vi "DataProcessorRAW.vi"(5 "FPGA in":refnum<queue>, 8 "Queue in":refnum<queue>) -> ()   [LabVIEW 2019, in "FPGA.lvlib"]
uses:
  FPGA.lvlib
  FPGA.ctl
  <vilib>/Analysis/baseanly.llb/Mean (DBL).vi
  <vilib>/Analysis/1siggen.llb/Ramp Pattern by Samples.vi
  ResultSweep.vi
  <vilib>/Analysis/NI_AALBase.lvlib
panel:
  in  "Save raw data":bool
  in  "Output from ADC (SW[9])":bool=TRUE
  in  "autoscale output signal":bool=TRUE
  out "Raw Data":ext[][](graph)
  in  "n. of steps":u32
  in  "Freq. slice start":dbl=10000.0
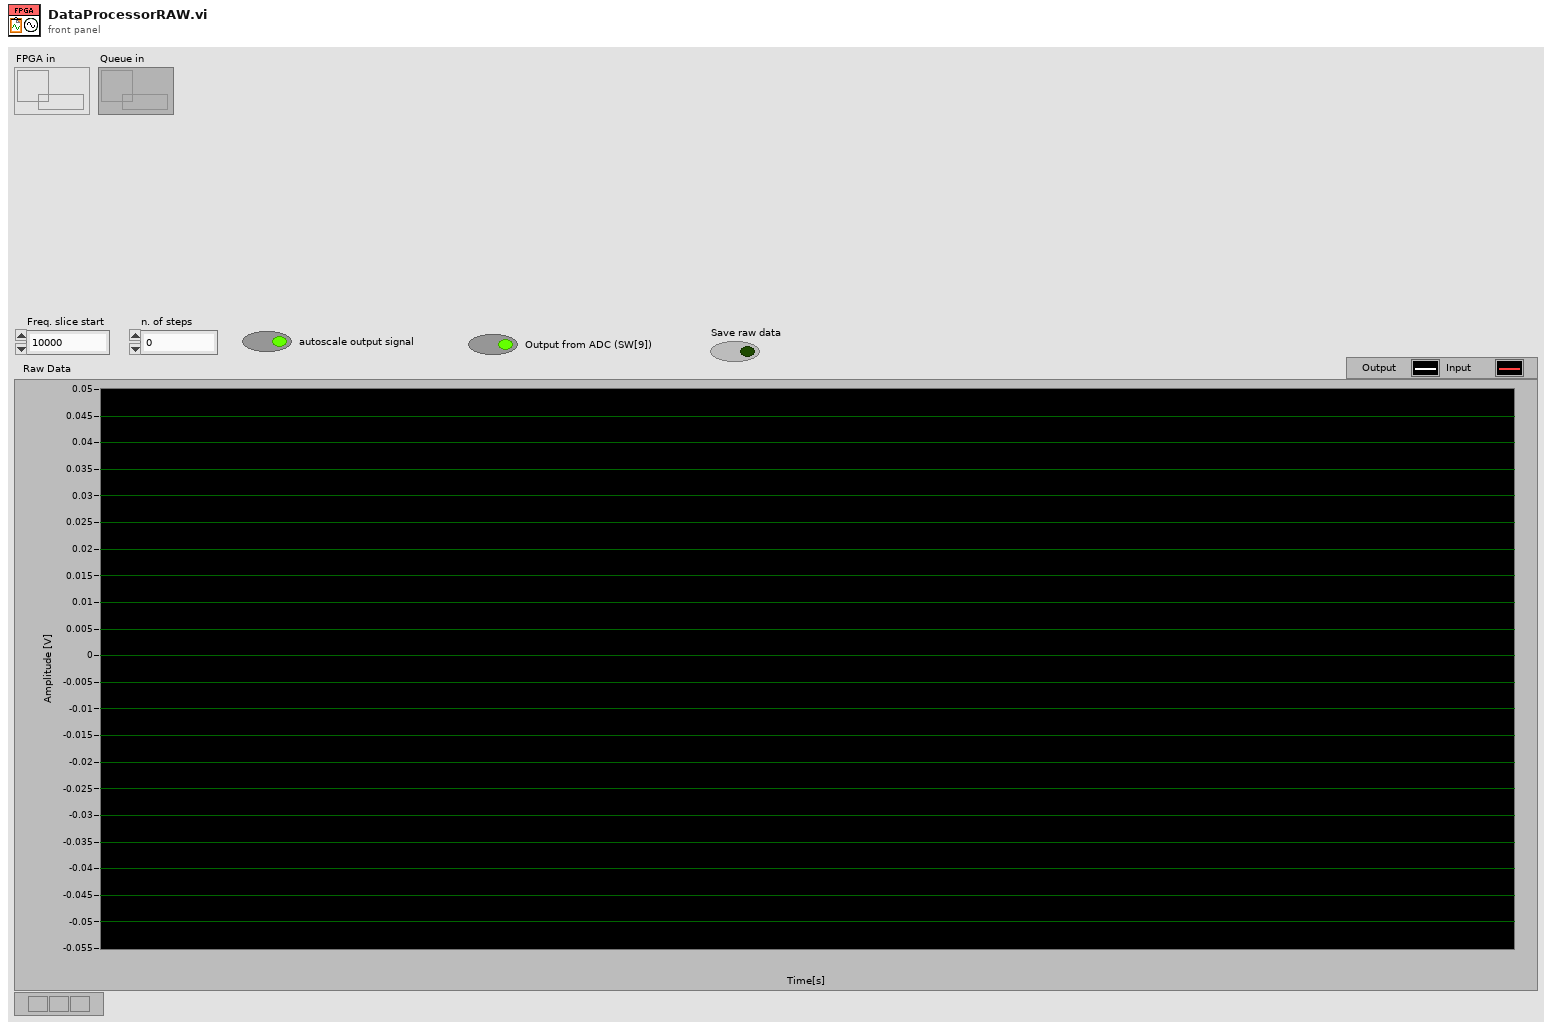
[diagram p1: front panel]
types:
  T1 = typedef "FPGA.lvlib/FPGA.ctl" = cluster{"Start freq. [Hz]":dbl, "Sweep duration [s]":dbl, "Freq. step [Hz]":dbl, "DAC Sample Rate":dbl, "ADC Sample Rate":dbl, "CMD port":u16, "DFAST port":u16, "CMD ID":refnum<k16>, "DFAST ID":refnum<k16>, "CMD error out":errorcluster, "FPGA IP":string, "DFAST error out ":errorcluster, "Stop freq. [Hz]":dbl, "Discrete sweep":bool, "Initial NCO":u32, "Difference NCO":i32, "step NCO":i64, "Final NCO":u32, "clocks for step":u32, "demodulation":bool, "NCO Phase Precision":u32, "NCO Sample Rate":dbl, "Time for step [s]":dbl, "NCO freq. resolution":dbl, "Sweep speed [Hz/s]":dbl, "Connected":bool, "Slew Rate [V/us]":dbl, "Parameters_ok":bool, "Amplitude [mVpp]":dbl, "Scale Factor":fxp<+,16,0>, "Acquiring":bool, "DAC-ADC Latency":u16, "Digital Gain":i32, "Number of steps":i32, "Averaging preferred":bool, "Filter Order":u32, "Settling":enum16{"99%", "99,9%"}}
  T2 = cluster{"Name":string, "Color":u32, "Style":u8, "Point Style":u8, "Name Visible":bool, "Allow Drag":bool, "Cursor Mode":u32, "Plot":i32, "Index":i32, "Position":cluster{"X":dbl, "Y":dbl}, "X Scale":u32, "Y Scale":u32, "Watch Plots":i32[], "Watch All Plots":bool, "Plot Area":i32, "Label Offset":cluster{"X":dbl, "Y":dbl}}
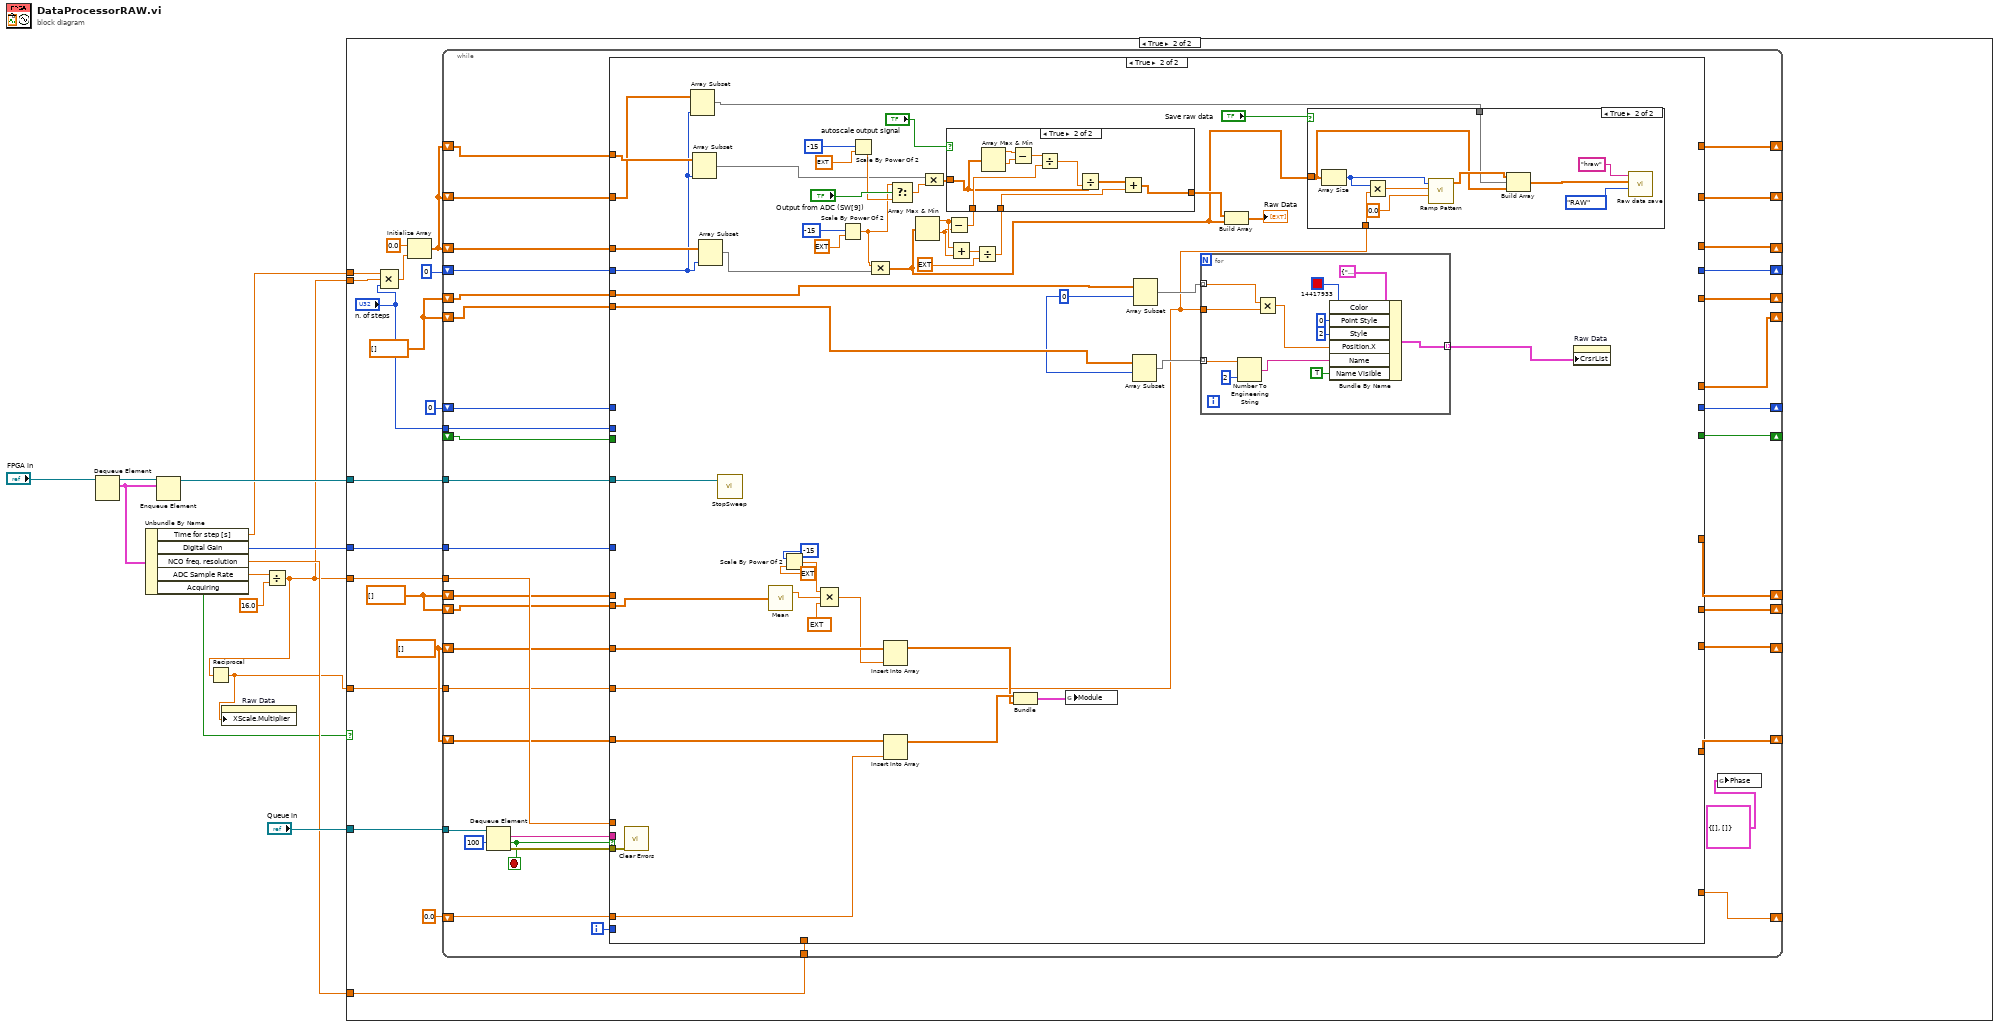
[diagram p0: block diagram]
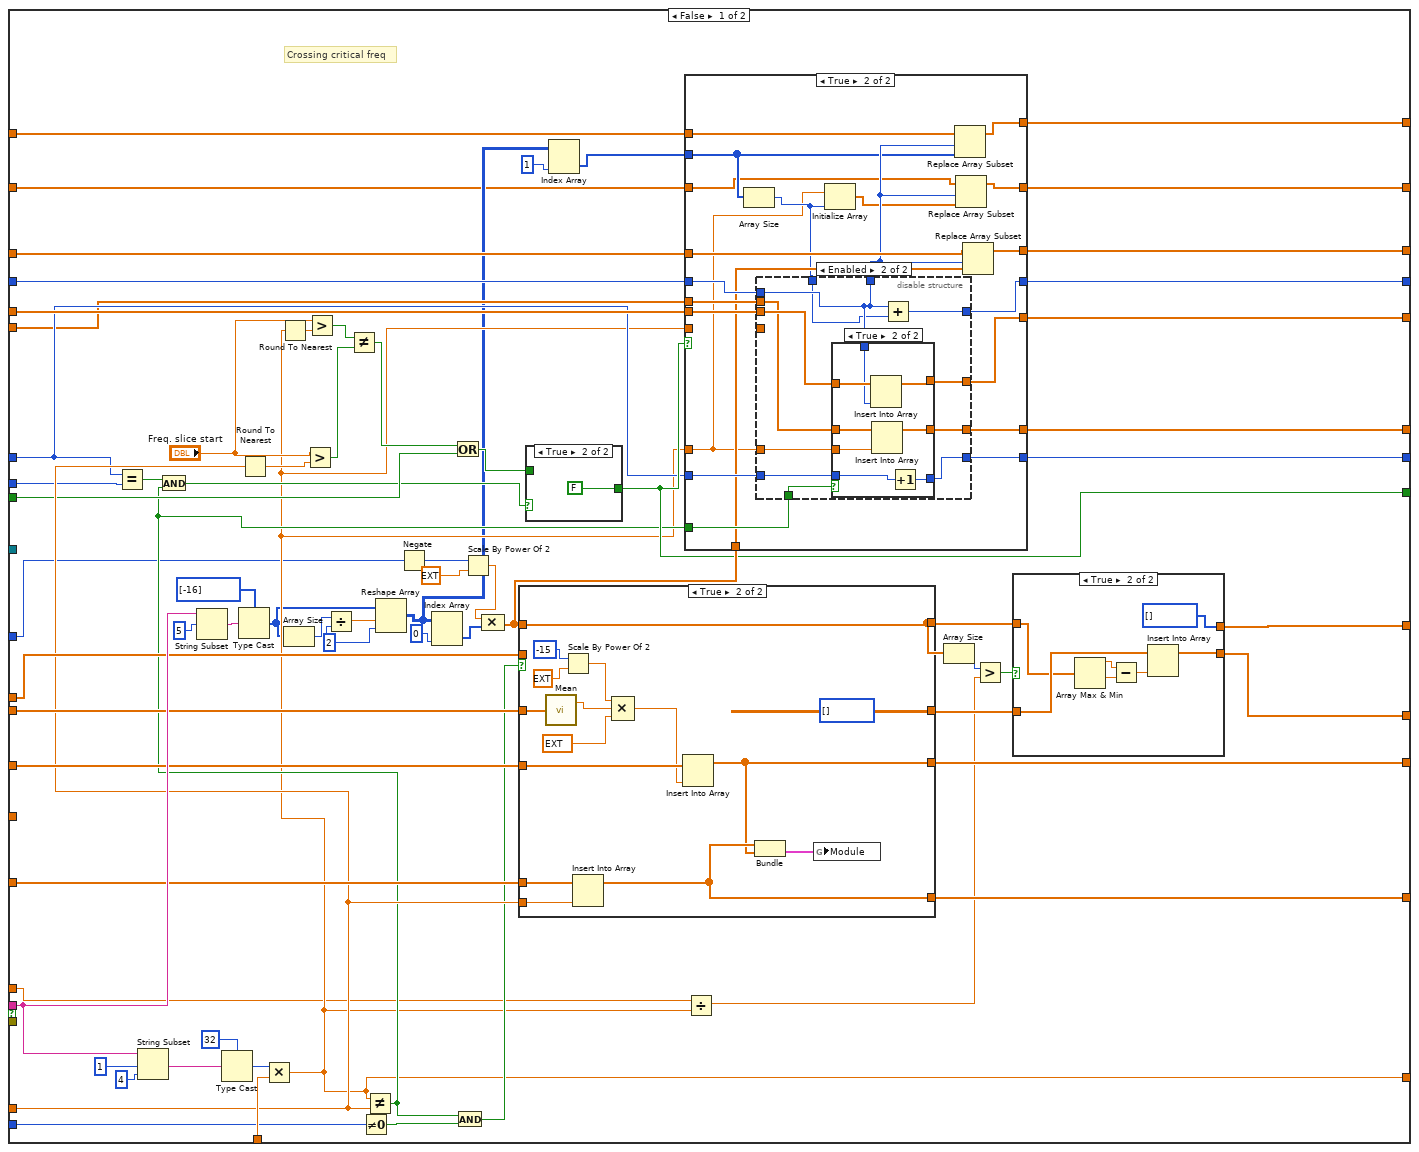
[diagram p3: hidden frame]
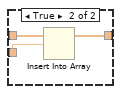
[diagram p7: hidden frame]
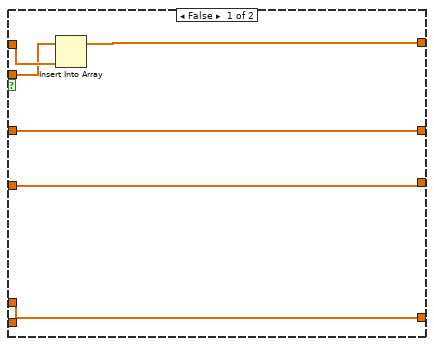
[diagram p10: hidden frame]
diagram:
  n1 = Dequeue Element(queue="FPGA in") -> (queue out=w7:refnum<queue>, element=w6:T1)  [unwired: 2 in, 2 out]
  n2 = Unbundle By Name(w6) -> ("Time for step [s]"=w2:dbl, "Digital Gain"=w4:i32, "NCO freq. resolution"=w11:dbl, "ADC Sample Rate"=w10:dbl, "Acquiring"=w8:bool)
  n3 = Enqueue Element(queue=w7, element=w6) -> (queue out=w5:refnum<queue>)  [unwired: 2 in, 2 out]
  n4 = Divide(x=w10, y=16.0) -> (x/y=w1:dbl)
  n5 = Reciprocal(x=w1) -> (1/x=w3:dbl)
  n6 = property on="Raw Data" class="WFGraph (strict)"("XScale.Multiplier"=w3) -> ()  [unwired: 2 in, 2 out]
  n7 = case shown="True" w8 {
    tunnel: w11 -> [_ w30]
    tunnel: "Queue in" -> [_ w31]
    tunnel: w1 -> [_ w29]
    tunnel: w5 -> [_ w26]
    tunnel: w4 -> [_ w25]
    tunnel: w3 -> [_ w23]
    tunnel: w2 -> [_ w18]
    tunnel: w1 -> [_ w17]
    frame False {
    }
    frame True {
      w15 = dbl[] []
      w27 = dbl[] []
      w22 = dbl[] []
      n8 = Compound Arithmetic op=MULTIPLY(w18, w17, "n. of steps") -> (w20:dbl)
      n9 = Initialize Array(0.0 ("element"), w20) -> (w14:dbl[])
      n10 = while {
        tunnel: w31 -> [w69]
        shift-right: [w62] -> _
        shift-left: 0.0 ("length (rest)") -> [w63]
        tunnel: w30 -> [w66]
        tunnel: w29 -> [w65]
        shift-right: [w59] -> _
        shift-left: w22 -> [w64]
        shift-right: [w60] -> _
        shift-left: w22 -> [w61]
        shift-right: [w57] -> _
        shift-left: w27 -> [w58]
        shift-right: [w54] -> _
        shift-left: w27 -> [w55]
        tunnel: w26 -> [w53]
        tunnel: w25 -> [w50]
        shift-right: [w48] -> _
        shift-left: w14 -> [w49]
        shift-right: [w46] -> _
        shift-left: w15 -> [w47]
        shift-right: [w45] -> _
        shift-left: _ -> [w44]
        shift-right: [w42] -> _
        shift-left: u32 0 -> [w43]
        tunnel: w23 -> [w41]
        shift-right: [w39] -> _
        shift-left: w15 -> [w40]
        tunnel: "n. of steps" -> [w38]
        shift-right: [w36] -> _
        shift-left: u32 0 -> [w37]
        shift-right: [w34] -> _
        shift-left: w14 -> [w35]
        shift-right: [w32] -> _
        shift-left: w14 -> [w33]
        i -> [w56]
        stop <- w52 stop-if-true
        n11 = Dequeue Element(queue=w69, timeout in ms (-1)=100) -> (element=w68:string, timed out?=w52:bool, error out=w67:errorcluster)  [unwired: 1 in, 1 out]
        n12 = case shown="True" w52 {
          tunnel: w68 -> [w138 _]
          tunnel: w67 -> [_ w279]
          tunnel: w66 -> [w135 _]
          tunnel: w65 -> [w85 _]
          tunnel: w64 -> [w134 _]
          tunnel: w63 -> [w112 w276]
          tunnel: [w86 _] -> w62
          tunnel: w61 -> [w131 w267]
          tunnel: [w133 _] -> w60
          tunnel: [w132 _] -> w59
          tunnel: w58 -> [w130 w278]
          tunnel: [w117 _] -> w57
          tunnel: w56 -> [w128 _]
          tunnel: w55 -> [w126 w277]
          tunnel: [w118 _] -> w54
          tunnel: w53 -> [_ w275]
          tunnel: w50 -> [w80 _]
          tunnel: w49 -> [w109 w238]
          tunnel: [w108 _] -> w48
          tunnel: w47 -> [w103 w261]
          tunnel: [w106 _] -> w46
          tunnel: [w99 _] -> w45
          tunnel: w44 -> [w104 _]
          tunnel: w43 -> [w96 _]
          tunnel: [w97 _] -> w42
          tunnel: w41 -> [_ w235]
          tunnel: w40 -> [w95 w260]
          tunnel: [w94 _] -> w39
          tunnel: w38 -> [w91 _]
          tunnel: w37 -> [w90 w231]
          tunnel: [w89 _] -> w36
          tunnel: w35 -> [w79 w240]
          tunnel: [w78 _] -> w34
          tunnel: w33 -> [w72 w233]
          tunnel: [w71 _] -> w32
          frame False {
            w75 = 2 ("dimension size")
            # "Crossing critical freq"
            n13 = Equal?(x=w96, y=w91) -> (x = y?=w102:bool)
            n14 = String Subset(string=w138, offset (0)=1, length (rest)=4 ("length (rest)")) -> (substring=w137:string)
            n15 = String Subset(string=w138, offset (0)=5) -> (substring=w123:string)  [unwired: 1 in]
            n16 = Type Cast(type=u32 32 ("length (rest)"), x=w137) -> (*(type *) &x=w129:u32)
            n17 = Type Cast(type=i16[] [-16], x=w123) -> (*(type *) &x=w84:i16[])
            n18 = Round To Nearest(number=w112) -> (nearest integer value=w92:dbl)
            n19 = Multiply(x=w129, y=w135) -> (x*y=w86:dbl)
            n20 = Round To Nearest(number=w86) -> (nearest integer value=w93:dbl)
            n21 = Array Size(array=w84) -> (size(s)=w83:i32)
            n22 = Greater?(x="Freq. slice start", y=w92) -> (0:w111:bool)
            n23 = Greater?(x="Freq. slice start", y=w93) -> (0:w110:bool)
            n24 = Divide(x=w83, y=w75) -> (x/y=w76:dbl)
            n25 = Not Equal?(x=w110, y=w111) -> (x != y?=w105:bool)
            n26 = Not Equal To 0?(x=w128) -> (x != 0?=w127:bool)
            n27 = Not Equal?(x=w86, y=w112) -> (x != y?=w88:bool)
            n28 = And(x=w102, y=w88) -> (x .and. y?=w101:bool)
            n29 = Reshape Array(w84, w76, w75) -> (w81:i16[][])
            n30 = Negate(x=w80) -> (-x=w114:i32)
            n31 = Index Array(array=w81, index (col)=0 ("index (row)")) -> (element=w82:i16[])  [unwired: 1 in]
            n32 = Or(x=w105, y=w104) -> (x .or. y?=w100:bool)
            n33 = And(x=w88, y=w127) -> (x .and. y?=w98:bool)
            n34 = Scale By Power Of 2(n=w114, x=ext 1.0) -> (x*2^n=w115:ext)
            n35 = Compound Arithmetic op=MULTIPLY(w115, w82) -> (w107:ext[])
            n36 = case shown="True" w98 {
              tunnel: [w215 w217] -> w119
              tunnel: w107 -> [w213 w217]
              tunnel: w134 -> [w212 _]
              tunnel: w131 -> [w214 w230]
              tunnel: [w214 i16[] []] -> w120
              tunnel: w130 -> [w211 w228]
              tunnel: [w211 w218] -> w117
              tunnel: w126 -> [w210 w227]
              tunnel: [w210 w225] -> w118
              tunnel: w112 -> [_ w226]
              frame False {
                n37 = Insert Into Array(array=w212, new element=w213) -> (w215:ext[])  [unwired: 1 in]
              }
              frame True {
                n38 = call-poly <vilib>:"Mean.vi"("X"=w230) -> ("mean"=w221:dbl)  [unwired: 1 out]
                n39 = Scale By Power Of 2(n=i16 -15, x=ext 1.0) -> (x*2^n=w222:ext)
                n40 = Insert Into Array(array=w227, new element=w226) -> (w225:dbl[])  [unwired: 1 in]
                n41 = Compound Arithmetic op=MULTIPLY(w222, w221, ext 1000.0 ("x")) -> (w219:ext)
                n42 = Insert Into Array(array=w228, new element=w219) -> (w218:dbl[])  [unwired: 1 in]
                n43 = Bundle(w225, w218) -> (w216:cluster{dbl[], dbl[]})  [unwired: 1 in]
                n44 = global write "ResultSweep.vi" "Module"(w216) -> ()
              }
            }
            n45 = case shown="True" w101 {
              tunnel: [w141 FALSE] -> w99
              tunnel: w100 -> [w141 _]
              frame False {
              }
              frame True {
              }
            }
            n46 = Index Array(array=w81, index (col)=1 ("index (row)")) -> (element=w77:i16[])  [unwired: 1 in]
            n47 = case shown="True" w99 {
              tunnel: w109 -> [w149 w160]
              tunnel: [w149 w161] -> w108
              tunnel: w107 -> [_ w159]
              tunnel: w103 -> [w148 w170]
              tunnel: [w148 w169] -> w106
              tunnel: w86 -> [_ _]
              tunnel: w88 -> [_ w168]
              tunnel: w96 -> [w147 w167]
              tunnel: [w147 w166] -> w97
              tunnel: w95 -> [w146 w165]
              tunnel: [w146 w164] -> w94
              tunnel: w86 -> [_ w153]
              tunnel: w90 -> [w145 w163]
              tunnel: [w145 w162] -> w89
              tunnel: w79 -> [w144 w158]
              tunnel: [w144 w157] -> w78
              tunnel: w77 -> [_ w155]
              tunnel: w72 -> [w143 w151]
              tunnel: [w143 w150] -> w71
              frame False {
              }
              frame True {
                n48 = Array Size(array=w155) -> (size(s)=w154:i32)
                n49 = disable-structure shown="Enabled" {
                  disable-tunnel: w170 -> [w174 w186]
                  disable-tunnel: [w173 w185] -> w169
                  disable-tunnel: _ -> [w172 _]
                  disable-tunnel: w168 -> [w171 w189]
                  disable-tunnel: w167 -> [_ w188]
                  disable-tunnel: [_ w187] -> w166
                  disable-tunnel: w165 -> [_ w184]
                  disable-tunnel: [_ w183] -> w164
                  disable-tunnel: w153 -> [_ w182]
                  disable-tunnel: w163 -> [_ w180]
                  disable-tunnel: [_ w181] -> w162
                  disable-tunnel: [_ w180] -> w156
                  disable-tunnel: w154 -> [_ w179]
                  frame Disabled {
                    n50 = case shown="False" w171 {
                      tunnel: w174 -> [w175 w178]
                      tunnel: [w175 w177] -> w173
                      tunnel: w172 -> [_ w176]
                      frame False {
                      }
                      frame True {
                        n51 = Insert Into Array(array=w178, new element=w176) -> (w177:dbl[])  [unwired: 1 in]
                      }
                    }
                  }
                  frame Enabled {
                    n52 = case shown="True" w189 {
                      tunnel: w188 -> [w192 w199]
                      tunnel: [w192 w200] -> w187
                      tunnel: w186 -> [w191 w198]
                      tunnel: [w191 w197] -> w185
                      tunnel: w184 -> [w190 w196]
                      tunnel: [w190 w195] -> w183
                      tunnel: w182 -> [_ w194]
                      tunnel: w180 -> [_ w193]
                      frame False {
                      }
                      frame True {
                        n53 = Insert Into Array(array=w198, new element=w193) -> (w197:dbl[])  [unwired: 1 in]
                        n54 = Insert Into Array(array=w196, new element=w194) -> (w195:dbl[])  [unwired: 1 in]
                        n55 = Increment(x=w199) -> (x+1=w200:u32)
                      }
                    }
                    n56 = Add(x=w180, y=w179) -> (x+y=w181:u32)
                  }
                }
                n57 = Initialize Array(w153, w154) -> (w152:dbl[])
                n58 = Replace Array Subset(array=w158, new element=w155, index=w156) -> (w157:dbl[])
                n59 = Replace Array Subset(array=w151, new element=w152, index=w156) -> (w150:dbl[])
                n60 = Replace Array Subset(array=w160, new element=w159, index=w156) -> (w161:dbl[])
              }
            }
            n61 = Divide(x=w85, y=w86) -> (x/y=w87:dbl)
            n62 = Array Size(array=w119) -> (size(s)=w122:i32)
            n63 = Greater?(x=w122, y=w87) -> (0:w121:bool)
            n64 = case shown="True" w121 {
              tunnel: w119 -> [w202 w204]
              tunnel: [w202 i16[] []] -> w132
              tunnel: w120 -> [w201 w209]
              tunnel: [w201 w208] -> w133
              frame False {
              }
              frame True {
                n65 = Array Max & Min(array=w204) -> (max value=w206:ext, min value=w205:ext)  [unwired: 2 out]
                n66 = Subtract(x=w206, y=w205) -> (x-y=w207:ext)
                n67 = Insert Into Array(array=w209, new element=w207) -> (w208:dbl[])  [unwired: 1 in]
              }
            }
          }
          frame True {
            w259 = 0 ("index")
            n68 = call <vilib>:"Clear Errors.vi"("error in (no error)"=w279) -> ()  [unwired: 5 in, 2 out]
            n69 = Array Subset(array=w233, length=w231) -> (w232:dbl[])  [unwired: 1 in]
            n70 = Array Subset(array=w240, length=w231) -> (w239:dbl[])  [unwired: 1 in]
            n71 = Array Subset(array=w238, length=w231) -> (w237:dbl[])  [unwired: 1 in]
            n72 = call "StopSweep.vi"("FPGA in"=w275) -> ()  [unwired: 10 in, 1 out]
            n73 = call-poly <vilib>:"Mean.vi"("X"=w267) -> ("mean"=w271:dbl)  [unwired: 1 out]
            n74 = Scale By Power Of 2(n=i16 -15, x=ext 1.0) -> (x*2^n=w272:ext)
            n75 = Compound Arithmetic op=MULTIPLY(w272, w271, ext 1000.0 ("x")) -> (w266:ext)
            n76 = Scale By Power Of 2(n=i16 -15, x=ext 1.0) -> (x*2^n=w241:ext)
            n77 = Scale By Power Of 2(n=i16 -15, x=ext 2.5) -> (x*2^n=w242:ext)
            n78 = Compound Arithmetic op=MULTIPLY(w241, w237) -> (w236:ext[])
            n79 = Insert Into Array(array=w278, new element=w266) -> (w273:dbl[])  [unwired: 1 in]
            n80 = Insert Into Array(array=w277, new element=w276) -> (w274:dbl[])  [unwired: 1 in]
            n81 = Select(t=w241, s="Output from ADC (SW[9])", f=w242) -> (s? t:f=w244:ext)
            n82 = Array Max & Min(array=w236) -> (max value=w249:ext, min value=w248:ext)  [unwired: 2 out]
            n83 = Compound Arithmetic op=MULTIPLY(w239, w244) -> (w253:ext[])
            n84 = Subtract(x=w249, y=w248) -> (x-y=w250:ext)
            n85 = Add(x=w249, y=w248) -> (x+y=w247:ext)
            n86 = Divide(x=w247, y=ext 2.0) -> (x/y=w245:ext)
            n87 = case shown="True" "autoscale output signal" {
              tunnel: w250 -> [_ w296]
              tunnel: w253 -> [w290 w295]
              tunnel: [w290 w292] -> w252
              tunnel: w245 -> [_ w291]
              frame False {
              }
              frame True {
                n88 = Array Max & Min(array=w295) -> (max value=w299:ext, min value=w298:ext)  [unwired: 2 out]
                n89 = Subtract(x=w299, y=w298) -> (x-y=w297:ext)
                n90 = Divide(x=w297, y=w296) -> (x/y=w294:ext)
                n91 = Divide(x=w295, y=w294) -> (x/y=w293:ext[])
                n92 = Add(x=w293, y=w291) -> (x+y=w292:ext[])
              }
            }
            n93 = Bundle(w274, w273) -> (w257:cluster{dbl[], dbl[]})  [unwired: 1 in]
            n94 = global write "ResultSweep.vi" "Module"(w257) -> ()
            n95 = Array Subset(array=w260, index=w259) -> (w258:dbl[])  [unwired: 1 in]
            n96 = Array Subset(array=w261, index=w259) -> (w262:dbl[])  [unwired: 1 in]
            n97 = for {
              tunnel: [w311] -> w263 mode=indexing
              tunnel: w262 -> [w308] mode=indexing
              tunnel: w235 -> [w309]
              tunnel: w258 -> [w303] mode=indexing
              n98 = Number To Engineering String(2:i16 2 ("precision (6)"), 4:w303) -> (0:w302:string)  [unwired: 2 in]
              n99 = Multiply(x=w308, y=w309) -> (x*y=w307:dbl)
              n100 = Bundle By Name(cluster=T2 {"Name"="", "Color"=0, "Style"=0, "Point Style"=0, "Name Visible"=FALSE, "Allow Drag"=FALSE, "Cursor Mode"=0, "Plot"=0, "Index"=0, "Position"={"X"=0.0, "Y"=0.0}, "X Scale"=0, "Y Scale"=0, "Watch Plots"=[], "Watch All Plots"=FALSE, "Plot Area"=0, "Label Offset"={"X"=0.0, "Y"=0.0}}, "Color"=u32 14417933, "Point Style"=u8 0, "Style"=u8 2, "Position.X"=w307, "Name"=w302, "Name Visible"=TRUE) -> (w311:T2)
            }
            n101 = Build Array(w252, w236) -> (→"Raw Data":ext[][])
            n102 = case shown="True" "Save raw data" {
              tunnel: w232 -> [_ w285]
              tunnel: w236 -> [_ w284]
              tunnel: w235 -> [_ w282]
              frame False {
              }
              frame True {
                n103 = Array Size(array=w284) -> (size(s)=w287:i32)
                n104 = Multiply(x=w287, y=w282) -> (x*y=w288:dbl)
                n105 = call-poly <vilib>:"Ramp Pattern.vi"("start"=0.0, "end"=w288, "samples"=w287) -> ("Ramp Pattern"=w286:dbl[])  [unwired: 7 in, 1 out]
                n106 = Build Array(w286, w285, w284) -> (w283:ext[][])
                n107 = call "Raw data save.vi"("Enum"=enum16{"LOCKIN", "RAW"}."RAW", "Input"=w283, "file format"="hraw") -> ()  [unwired: 9 in]
              }
            }
            n108 = property on="Raw Data" class="WFGraph (strict)"("CrsrList"=w263) -> ()  [unwired: 2 in, 2 out]
          }
        }
        n109 = global write "ResultSweep.vi" "Phase"(cluster{dbl[], dbl[]} {[], []} ("output cluster")) -> ()
      }
    }
  }
